vi "testnotifier.vi"() -> ()   [LabVIEW 2018]
panel:
  out "c":dbl
  in  "b":dbl
  in  "a":dbl
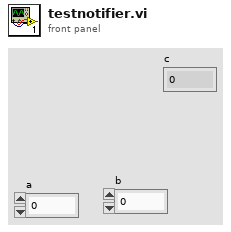
[diagram p1: front panel]
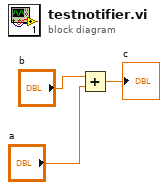
[diagram p0: block diagram]
diagram:
  n1 = Add(x="b", y="a") -> (x+y=→"c":dbl)
